vi "Create UDP Service.vi"(8 "error in (no error)":errorcluster, 10 "Service Details":T1, 11 "Main Display in":refnum<class "Main Display.lvclass">) -> (0 "error out":errorcluster, 3 "Main Display out":refnum<class "Main Display.lvclass">)   [LabVIEW 2016, in "Assert API Components.lvlib" / "Assert Display.lvlib" / "Main Display.lvlib" / "Main Display.lvclass"]
uses:
  Main Display.lvclass
  C:/Program Files (x86)/National Instruments/LabVIEW 2016/vi.lib/ActorFramework/Actor/Actor.lvclass
  Service Config Display/Service Config Display/Service Details.ctl
  UDP Service/UDP Service/UDP Service.lvclass
  Main Display.lvclass/Main Display.ctl
  UDP Service/UDP Service/UDP Service.lvclass/UDP Service.ctl
  <vilib>/ActorFramework/Actor/Actor.lvclass
  Assert Display/Assert Display.lvlib
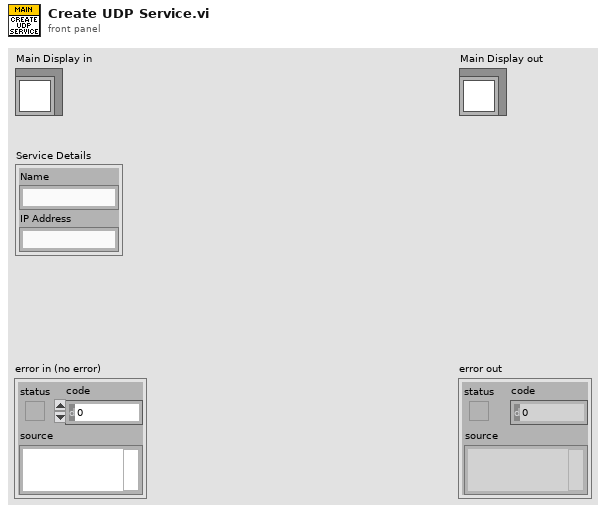
[diagram p1: front panel]
types:
  T1 = typedef "Assert API Components.lvlib/Assert Display.lvlib/Service Details.ctl" = cluster{"Name":string, "IP Address":string}
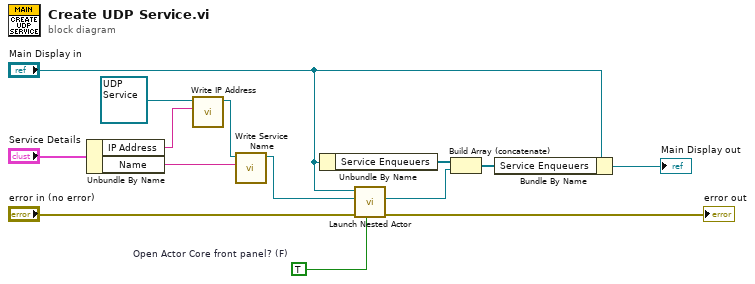
[diagram p0: block diagram]
diagram:
  w1 = TRUE  # Open Actor Core front panel? (F)
  n1 = Unbundle By Name("Service Details") -> ("IP Address"=w11:string, "Name"=w2:string)
  n2 = call "Write IP Address.vi"("IP Address"=w11, "UDP Service in"=refnum<class "UDP Service.lvclass"> refnum ("UDP Service.lvlib:UDP Service.lvclass")) -> ("UDP Service out"=w9:refnum<class "UDP Service.lvclass">)  [unwired: 9 in]
  n3 = call "Write Service Name.vi"("Service Name"=w2, "UDP Service in"=w9) -> ("UDP Service out"=w8:refnum<class "UDP Service.lvclass">)  [unwired: 9 in]
  n4 = Unbundle By Name("Main Display in") -> ("Service Enqueuers"=w5:refnum<class "Message Enqueuer.lvclass">[])
  n5 = call <vilib>:"Launch Nested Actor.vi"("Open Actor Core front panel? (F)"=w1, "error in (no error)"="error in (no error)", "Nested Actor"=w8, "Caller Actor in"="Main Display in") -> ("error out"=→"error out":errorcluster, "Nested Actor's Enqueuer"=w4:refnum<class "Message Enqueuer.lvclass">)  [unwired: 5 in, 1 out]
  n6 = Build Array (concatenate)(w5, w4) -> (w3:refnum<class "Message Enqueuer.lvclass">[])
  n7 = Bundle By Name(cluster="Main Display in", "Service Enqueuers"=w3) -> (→"Main Display out":refnum<class "Main Display.lvclass">)
